vi "HexToNormalString.vi"(7 "Hex Display":string="\u0001") -> (8 "Normal Display":string)   [LabVIEW 2015]
doc: "This VI translate the hex display string to normal display string. The two type string display the same."
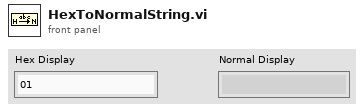
[diagram p1: front panel]
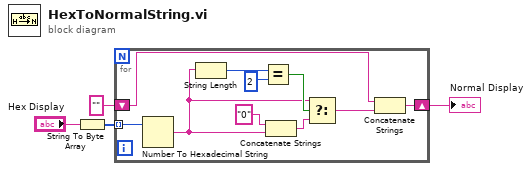
[diagram p0: block diagram]
diagram:
  n1 = String To Byte Array(string="Hex Display") -> (unsigned byte array=w2:u8[])
  n2 = for {
    tunnel: w2 -> [w14] mode=indexing
    shift-right: [w13] -> w3
    shift-left: "" -> [w12]
    n3 = Number To Hexadecimal String(2:w14) -> (0:w7:string)  [unwired: 1 in]
    n4 = String Length(string=w7) -> (length=w11:i32)
    n5 = Equal?(x=w11, y=2) -> (x = y?=w9:bool)
    n6 = Concatenate Strings("0" ("字符串"), w7) -> (w5:string)
    n7 = Select(t=w7, s=w9, f=w5) -> (s? t:f=w8:string)
    n8 = Concatenate Strings(w12, w8) -> (w13:string)
  }
  "Normal Display" <- w3
